vi "Testing 8SCP to 16SPC converter.vi"() -> ()   [LabVIEW 2015]
uses:
  <instrlib>/_niInstr/Basic Elements/v1/FPGA/Private/Count Down U16.vi
  <instrlib>/_niInstr/Basic Elements/v1/FPGA/Private/Count Up U16.vi
  DDC_7976R_v1.lvlib
  <vilib>/Analysis/NI_AALBase.lvlib
  <instrlib>/_niInstr/Basic Elements/v1/FPGA/niInstr Basic Elements v1 FPGA.lvlib
panel:
  out "Total iterations":i32
  out "size(s)":i32[](array[numeric])
  out "size":i32
  in  "element":dbl format="%#_13g"
  out "appended array":dbl[][](graph)
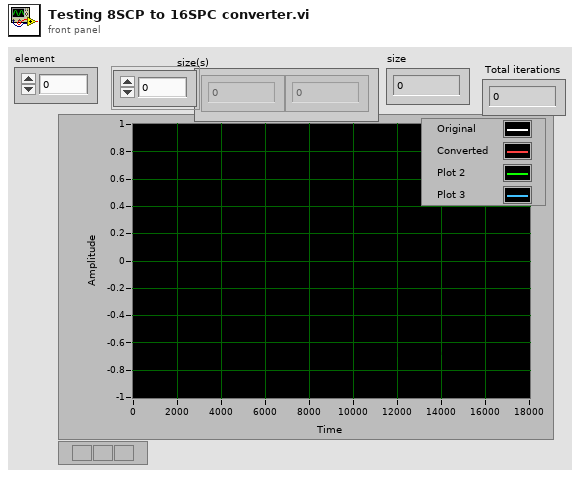
[diagram p1: front panel]
types:
  T1 = typedef "niInstr DSP v1 Shared.lvlib/IQ Data.ctl" = cluster{"I":fxp<+/-,18,1>, "Q":fxp<+/-,18,1>, "overflow":bool}
  T2 = typedef "DDC_7976R_v1.lvlib/16xIQData.ctl" = T1[]
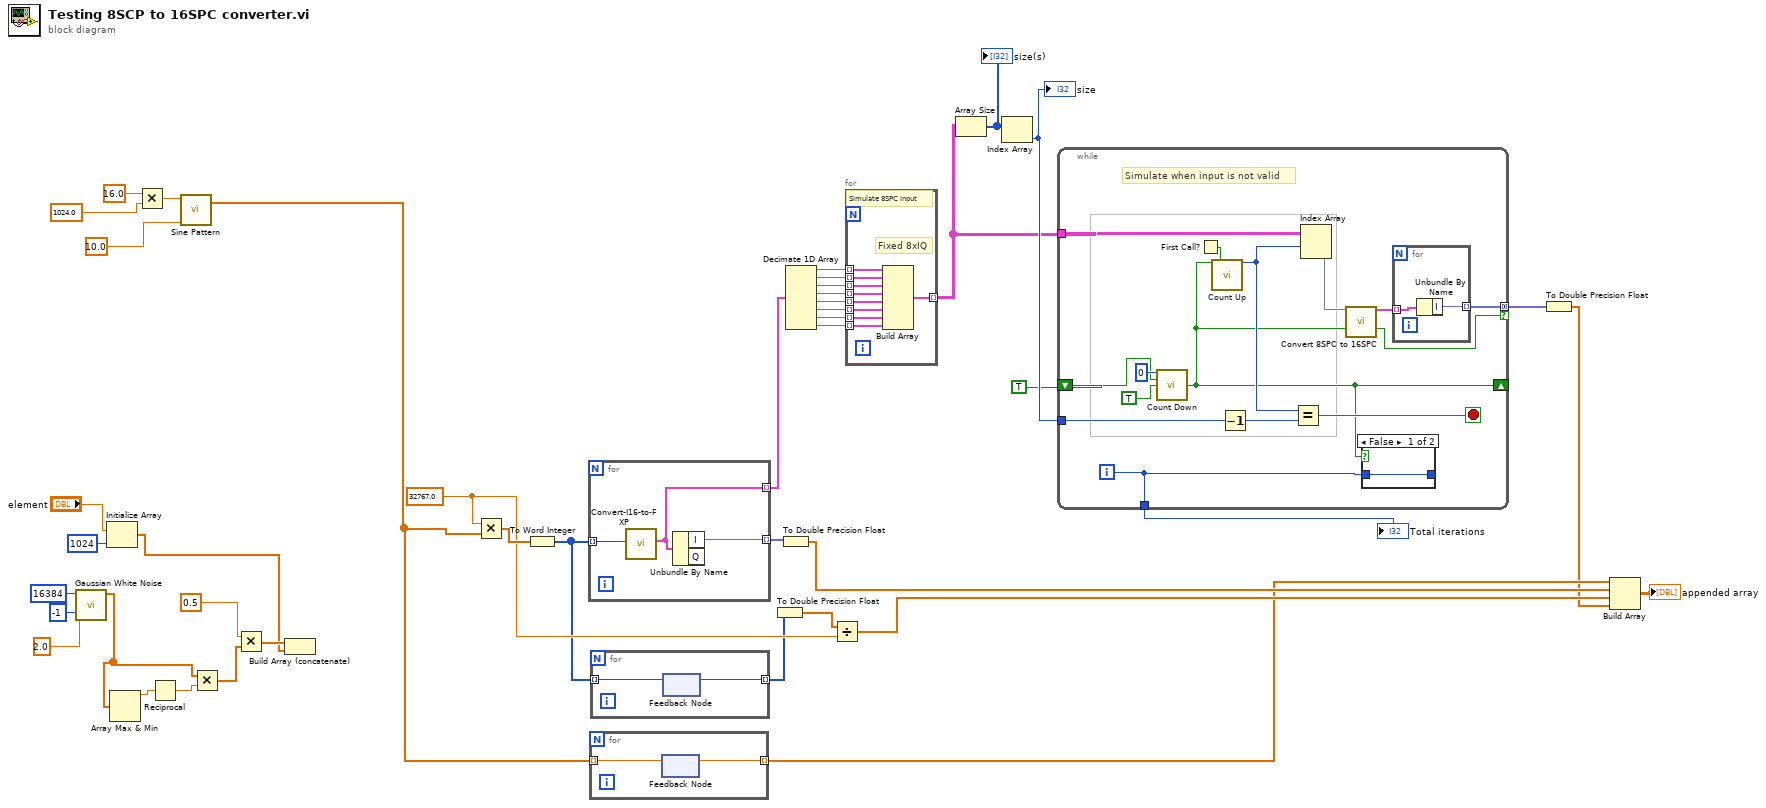
[diagram p0: block diagram]
diagram:
  w31 = 32767.0
  n1 = call <vilib>:"Gaussian White Noise.vi"("seed"=-1, "standard deviation"=2.0, "samples"=16384) -> ("Gaussian noise pattern"=w38:dbl[])  [unwired: 7 in, 1 out]
  n2 = Initialize Array("element", 1024 ("dimension size")) -> (w26:dbl[])
  n3 = Array Max & Min(array=w38) -> (max value=w39:dbl)  [unwired: 3 out]
  n4 = Multiply(x=16.0, y=1024.0) -> (x*y=w21:dbl)
  n5 = Reciprocal(x=w39) -> (1/x=w37:dbl)
  n6 = call <vilib>:"Sine Pattern.vi"("cycles"=10.0, "samples"=w21) -> ("Sinusoidal Pattern"=w17:dbl[])  [unwired: 2 in, 1 out]
  n7 = Multiply(x=w38, y=w37) -> (x*y=w36:dbl[])
  n8 = Multiply(x=0.5, y=w36) -> (x*y=w27:dbl[])
  n9 = Build Array (concatenate)(w27, w26) -> ()  [unwired: 1 out]
  n10 = Multiply(x=w31, y=w17) -> (x*y=w35:dbl[])
  n11 = To Word Integer(number=w35) -> (16bit integer=w23:i16[])
  n12 = for {
    tunnel: w23 -> [w46] mode=indexing
    tunnel: [w45] -> w34 mode=indexing
    tunnel: [w44] -> w16 mode=indexing
    n13 = call "Convert-I16-to-FXP.vi"("I16 in"=w46) -> ("data out"=w44:T1)  [unwired: 6 in]
    n14 = Unbundle By Name(w44) -> ("I"=w45:fxp<+/-,18,1>)  [unwired: 1 out]
  }
  n15 = for {
    tunnel: w17 -> [w48] mode=indexing
    tunnel: [w47] -> w24 mode=indexing
    n16 = feedback #1() -> (w47:dbl)  [unwired: 1 in]
    n17 = feedback-in #1(w48) -> ()
  }
  n18 = for {
    tunnel: w23 -> [w50] mode=indexing
    tunnel: [w49] -> w22 mode=indexing
    n19 = feedback #2() -> (w49:i16)  [unwired: 1 in]
    n20 = feedback-in #2(w50) -> ()
  }
  n21 = To Double Precision Float(number=w22) -> (double precision float=w32:dbl[])
  n22 = To Double Precision Float(number=w34) -> (double precision float=w25:dbl[])
  n23 = Decimate 1D Array(w16) -> (w15:T1[], w14:T1[], w13:T1[], w12:T1[], w11:T1[], w10:T1[], w9:T1[], w8:T1[])
  n24 = Divide(x=w32, y=w31) -> (x/y=w30:dbl[])
  n25 = for {
    tunnel: w15 -> [w59] mode=indexing
    tunnel: w14 -> [w58] mode=indexing
    tunnel: w13 -> [w57] mode=indexing
    tunnel: w12 -> [w56] mode=indexing
    tunnel: w11 -> [w55] mode=indexing
    tunnel: w10 -> [w54] mode=indexing
    tunnel: w9 -> [w53] mode=indexing
    tunnel: w8 -> [w52] mode=indexing
    tunnel: [w51] -> w3 mode=indexing
    # "Fixed 8xIQ"
    # "Simulate 8SPC input"
    n26 = Build Array(w59, w58, w57, w56, w55, w54, w53, w52) -> (w51:T1[])
  }
  n27 = Array Size(array=w3) -> (size(s)=w6:i32[])
  "size(s)" <- w6
  n28 = Index Array(array=w6) -> (element=w4:i32)  [unwired: 1 in]
  "size" <- w4
  n29 = while {
    tunnel: [w73] -> w5 mode=concatenating if=w74
    shift-right: [w61] -> _
    shift-left: TRUE ("decrement") -> [w70]
    tunnel: w4 -> [w67]
    tunnel: w3 -> [w64]
    tunnel: [w60] -> w2
    i -> [w60]
    stop <- w65 stop-if-true
    # "Simulate when input is not valid"
    n30 = call-poly <instrlib>:"Count Down.vi"("count in"=u16 0, "load"=w70, "decrement"=TRUE) -> ("terminal count"=w61:bool)  [unwired: 11 in, 1 out]
    n31 = First Call?() -> (First Call?: T/F=w68:bool)
    n32 = call-poly <instrlib>:"Count Up.vi"("increment"=w61, "reset"=w68) -> ("count out"=w63:u16)  [unwired: 13 in]
    n33 = Decrement(x=w67) -> (x-1=w66:i32)
    n34 = Equal?(x=w63, y=w66) -> (x = y?=w65:bool)
    n35 = Index Array(array=w64, index (row)=w63) -> (element=w62:T1[])  [unwired: 1 in]
    n36 = call "Convert 8SPC to 16SPC.vi"("8xIQ in"=w62, "input valid"=w61) -> ("16xIQ out"=w69:T2, "output valid"=w74:bool)  [unwired: 12 in]
    n37 = case shown="False" w61 {
      tunnel: w60 -> [w75 w76]
      tunnel: [w75 w76] -> _
      frame False {
      }
      frame True {
      }
    }
    n38 = for {
      tunnel: w69 -> [w78] mode=indexing
      tunnel: [w77] -> w73 mode=indexing
      n39 = Unbundle By Name(w78) -> ("I"=w77:fxp<+/-,18,1>)
    }
  }
  "Total iterations" <- w2
  n40 = To Double Precision Float(number=w5) -> (double precision float=w7:dbl[])
  n41 = Build Array(w24, w25, w30, w7) -> (→"appended array":dbl[][])
